vi "Check Previous Values.vi"(8 "error in":errorcluster, 10 "values":dbl[](array[numeric]), 11 "Tx Execution Unit Implementation in":refnum<class "Tx Execution Unit.lvclass">) -> (0 "error out":errorcluster, 1 "values modified?":bool, 2 "values out":dbl[](array[numeric]), 3 "Tx Execution Unit Implementation out":refnum<class "Tx Execution Unit.lvclass">)   [LabVIEW 2021, in "Ballard MIL-STD-1553 Engine.lvlib" / "Implementation.lvlib" / "Tx Execution Unit.lvclass"]
uses:
  Tx Execution Unit.lvclass
  Tx Execution Unit.lvclass/Tx Execution Unit.ctl
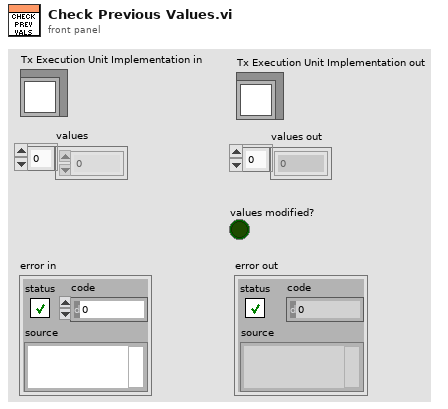
[diagram p1: front panel]
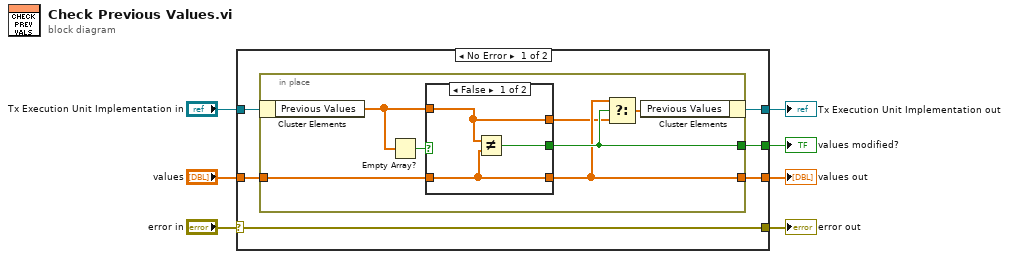
[diagram p0: block diagram]
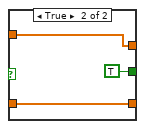
[diagram p2: hidden frame]
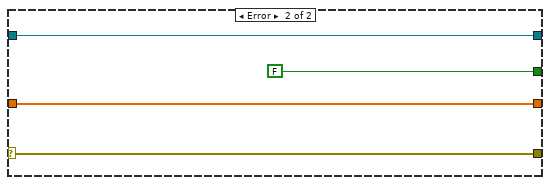
[diagram p3: hidden frame]
diagram:
  n1 = case shown="No Error" "error in" {
    selector: "error in" -> [w11 w27]
    tunnel: [w13 FALSE] -> w7
    tunnel: [w12 w28] -> w6
    tunnel: [w8 w30] -> w5
    tunnel: "Tx Execution Unit Implementation in" -> [w9 w30]
    tunnel: "values" -> [w10 w28]
    tunnel: [w11 w27] -> w1
    frame No Error {
      n2 = in-place {
        in-place-border: [w19] -> w13
        in-place-border: [w15] -> w12
        in-place-border: w10 -> [w20]
        n3 = in-place-cluster #1(w9) -> ("Previous Values"=w17:dbl[])
        n4 = Empty Array?(array=w17) -> (empty?=w16:bool)
        n5 = case shown="False" w16 {
          tunnel: w20 -> [w22 w25]
          tunnel: [w21 TRUE] -> w19
          tunnel: w17 -> [w23 w24]
          tunnel: [w22 w25] -> w15
          tunnel: [w23 w24] -> w14
          frame False {
            n6 = Not Equal?(x=w23, y=w22) -> (x != y?=w21:bool)
          }
          frame True {
          }
        }
        n7 = Select(t=w15, s=w19, f=w14) -> (s? t:f=w18:dbl[])
        n8 = in-place-cluster #1("Previous Values"=w18) -> (w8:refnum<class "Tx Execution Unit.lvclass">)
      }
    }
    frame Error {
    }
  }
  "values out" <- w6
  "values modified?" <- w7
  "Tx Execution Unit Implementation out" <- w5
  "error out" <- w1
